vi "Get ISO Time.vi"(8 "error in":errorcluster, 11 "LogRecord in":refnum<class "LogRecord.lvclass">) -> (0 "error out":errorcluster, 2 "ISO Time":string, 3 "LogRecord out":refnum<class "LogRecord.lvclass">)   [LabVIEW 2016, in "hse-logger.lvlib" / "LogRecord.lvclass"]
doc: "Returns the ISO-8601 formatted time of the LogRecord. \n\nDefault is with milliseconds.\n\n____\n(c) HAMPEL SOFTWARE ENGINEERING"
uses:
  LogRecord.lvclass
  LogRecord.lvclass/LogRecord.ctl
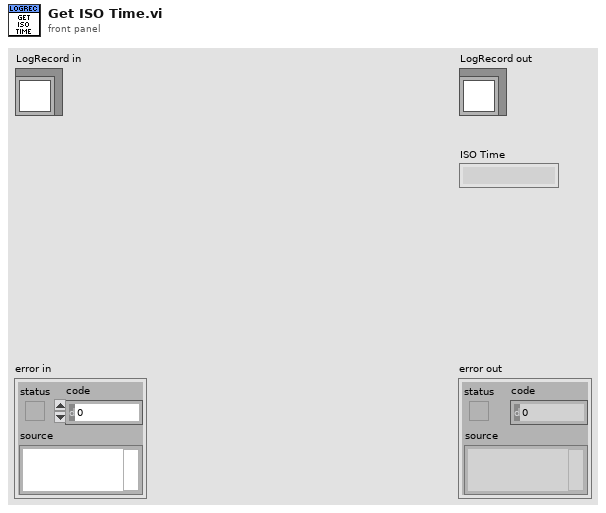
[diagram p1: front panel]
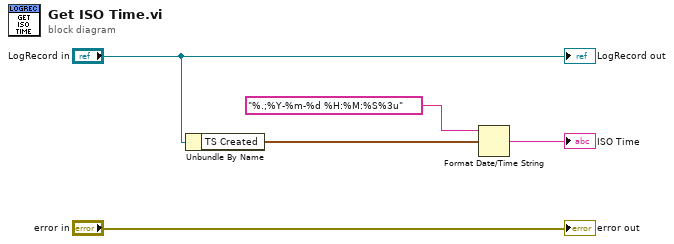
[diagram p0: block diagram]
diagram:
  n1 = Unbundle By Name("LogRecord in") -> ("TS Created"=w2:timestamp)
  n2 = Format Date/Time String(time format string (%c)="%.;%Y-%m-%d %H:%M:%S%3u", seconds (now)=w2) -> (date/time string=→"ISO Time":string)  [unwired: 1 in]
  "error out" <- "error in"
  "LogRecord out" <- "LogRecord in"
